vi "Dipper Fridge Resistance Measurement 1.3.vi"() -> ()   [LabVIEW 2011]
uses:
  <vilib>/express/express arith-compare/Formula/XNode/ExpressFormulaBlockNode.xnode
panel:
  out "He Pot Temperature":cluster{dbl[], dbl[]}(graph)
  out "Sample Resistance":dbl[][](graph)
  in  "Sample":bool
  out "Thermometer":bool
  out "Sample":bool
  in  "Timer":bool caption="Reset"
  out "Time Elapsed":string
  out "Output Power":dbl[unit]
  out "Heater Power (%)":string
  in  "Save":bool
  out "var":i32
  in  "error in (no error) 2":errorcluster
  in  "Output Range":string(combo)
  in  "Heater Power (%)":dbl caption="y"
  out "Heater Type (in Ohm)":string
  out "Heater Current (in %)":string
  out "Heater":bool
  in  "Heater":bool
  out "Boolean":bool
  in  "Power":bool
  in  "Date format (0)":enum16{"short", "long", "abbreviated"}(ring)
  out "Thermometer A":cluster{dbl[], dbl[unit][]}(graph)
  out "size (in bytes)":i64
  out "Thermometer (Ge17035)":cluster{dbl[], dbl[]}(graph)
  out "Warning":string="Can't be smaller than 1 s"
  in  "File Path":path
  out "current time":timestamp
  out "Number of Data points":i32
  in  "Time delay":u32=500 min=500 max=10000
  in  "error in (no error)":errorcluster
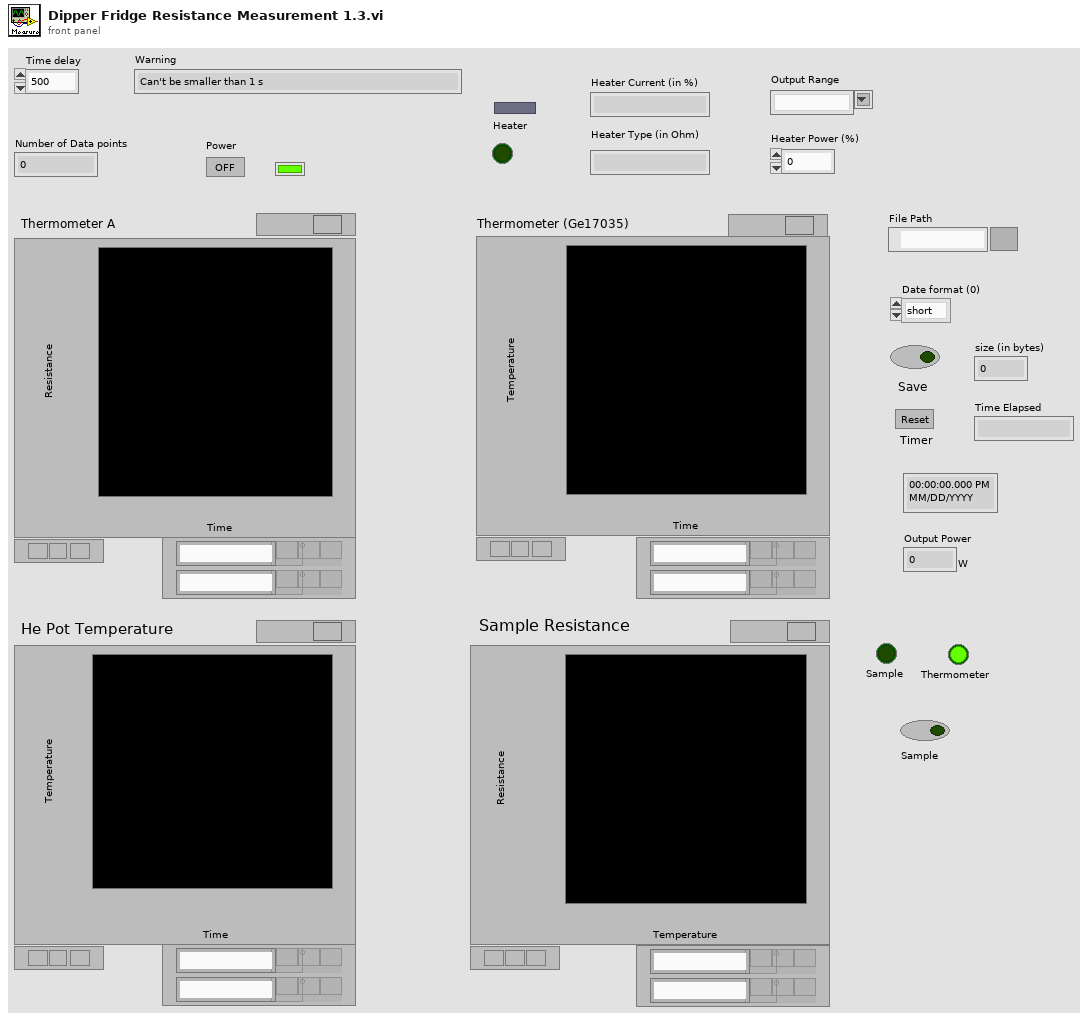
[diagram p1: front panel]
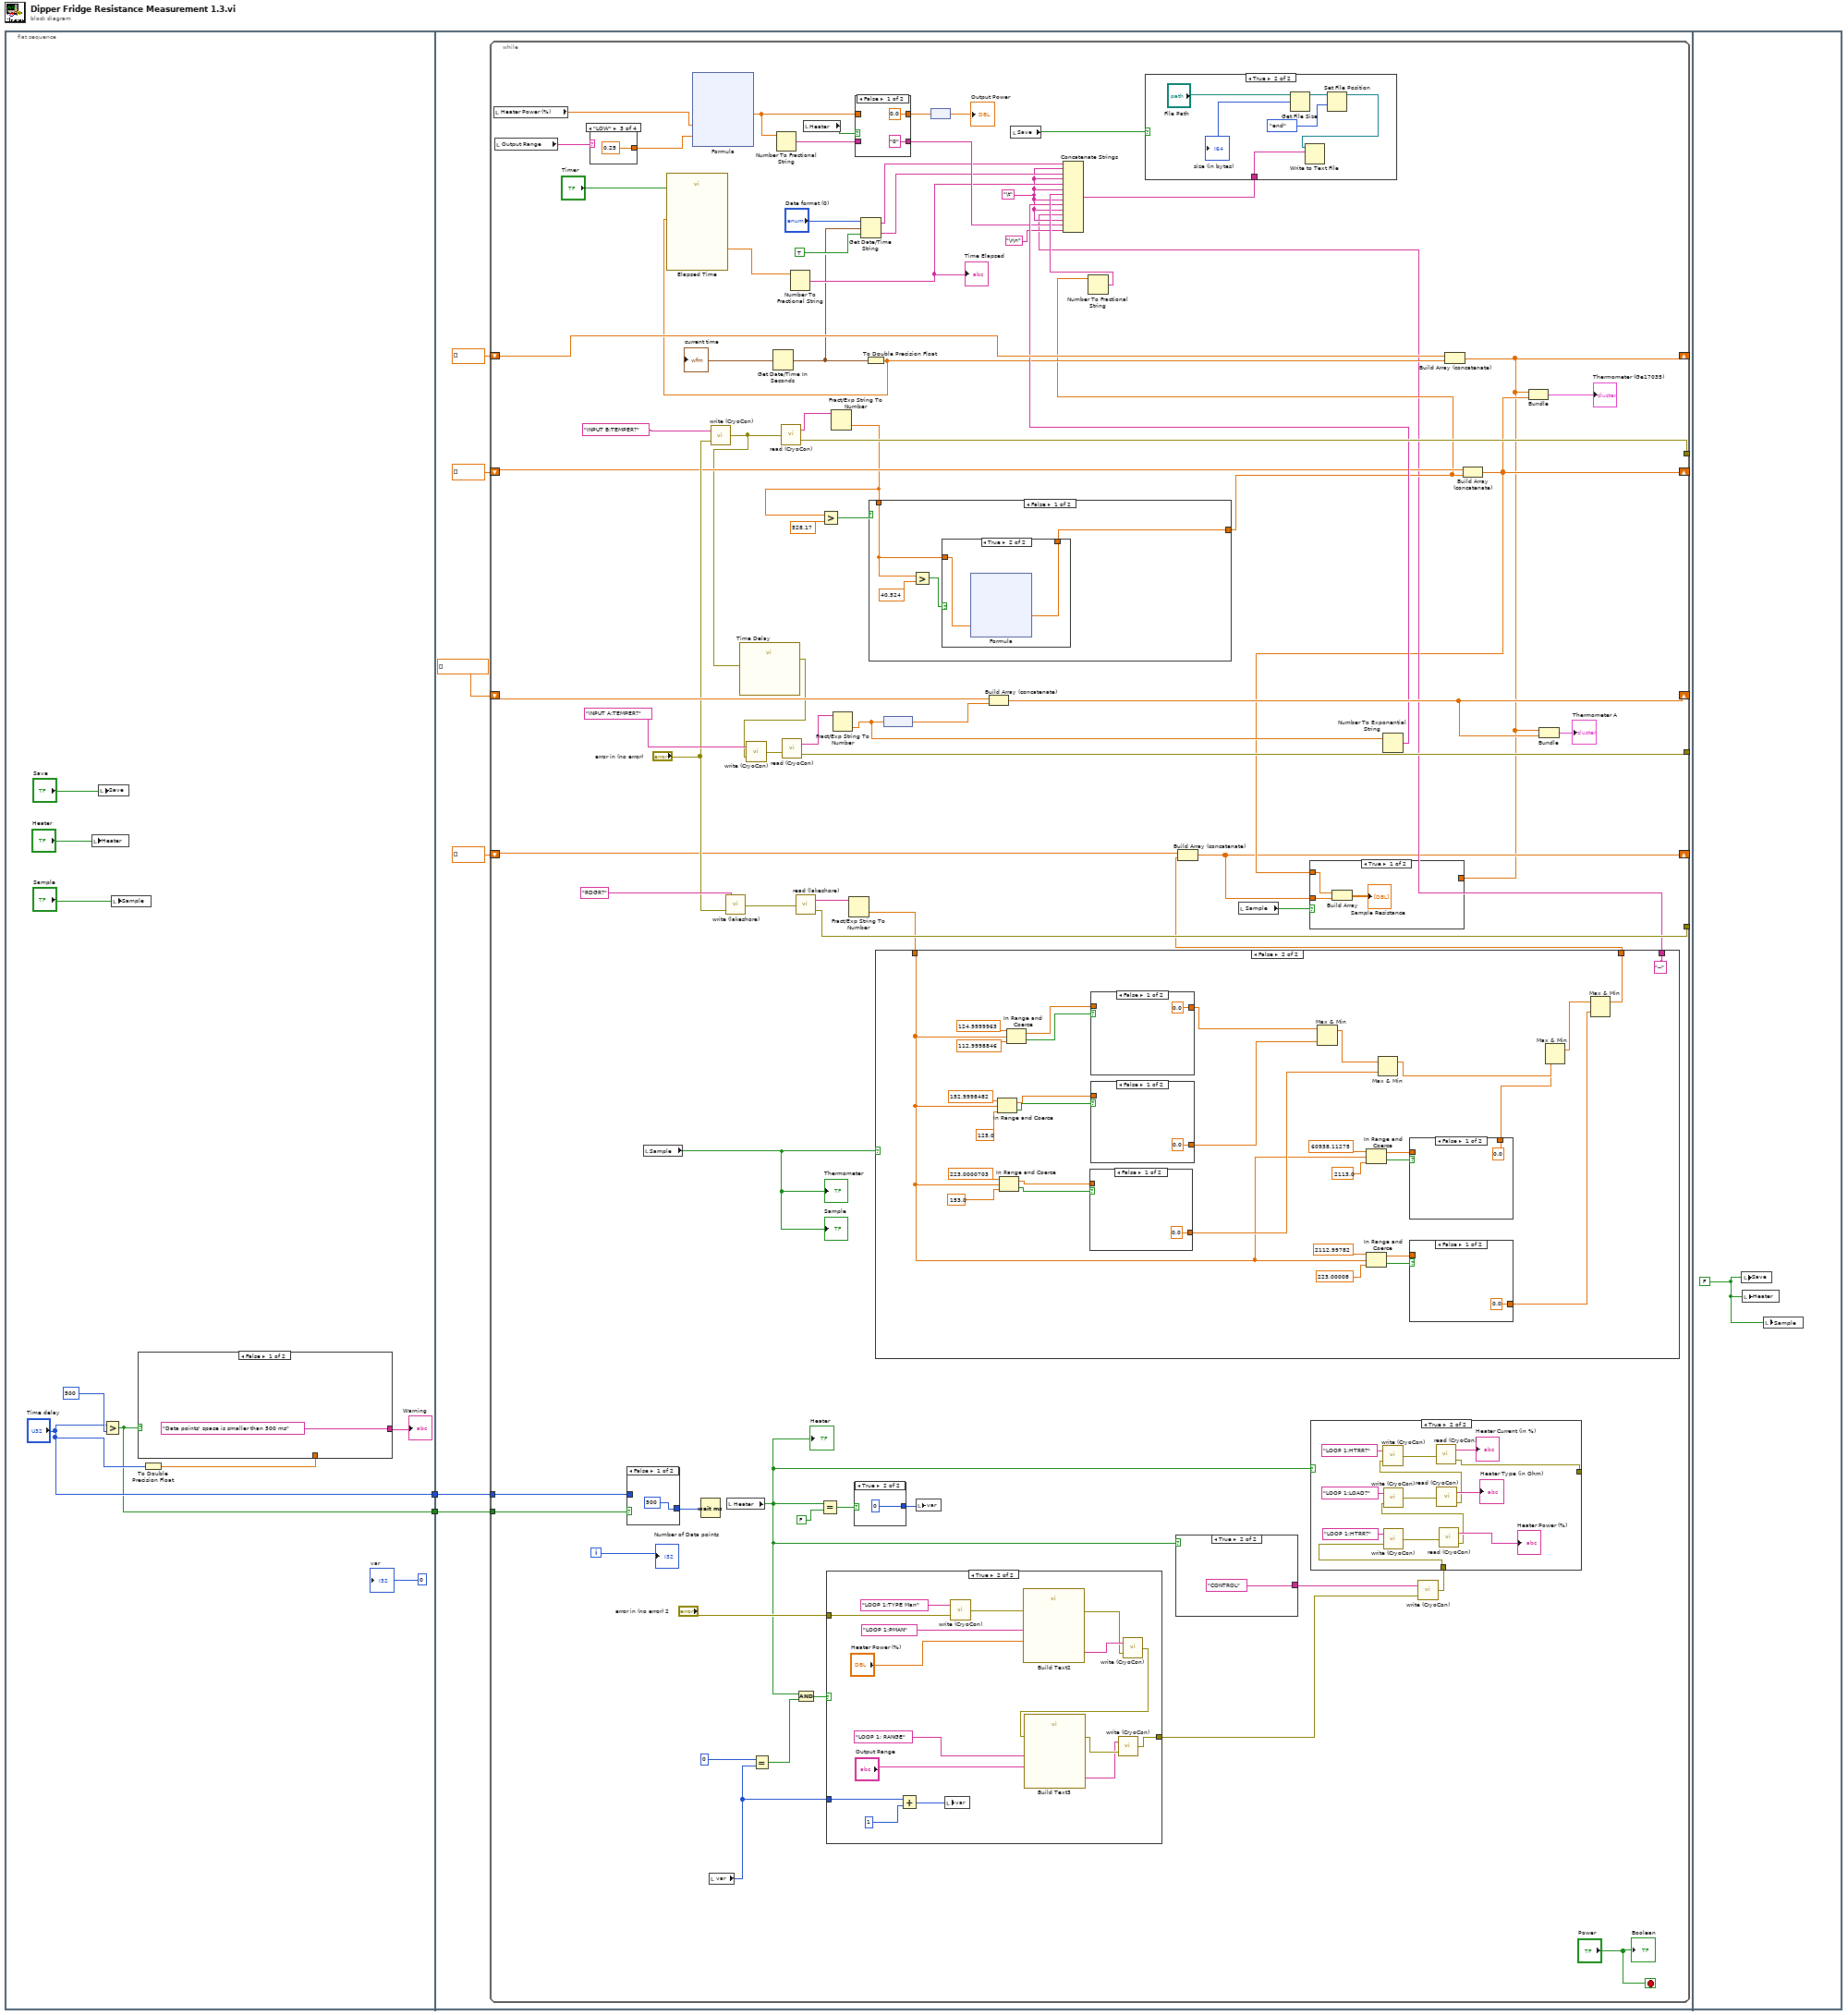
[diagram p0: block diagram]
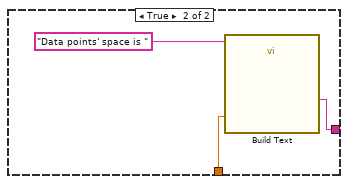
[diagram p2: hidden frame]
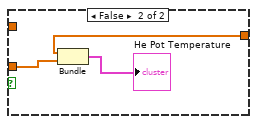
[diagram p3: hidden frame]
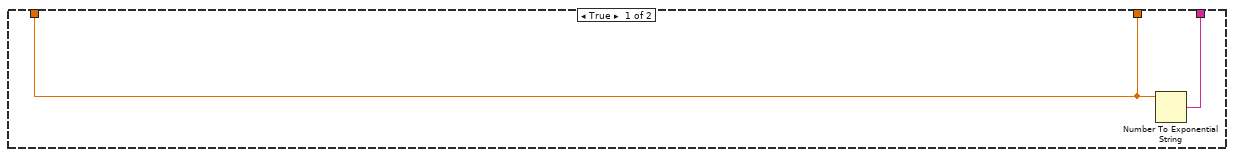
[diagram p4: hidden frame]
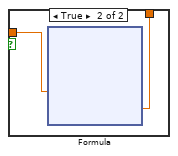
[diagram p5: hidden frame]
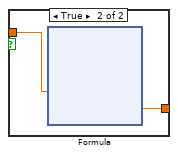
[diagram p6: hidden frame]
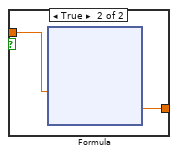
[diagram p7: hidden frame]
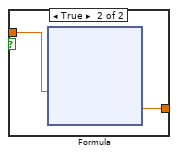
[diagram p8: hidden frame]
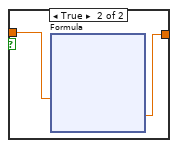
[diagram p9: hidden frame]
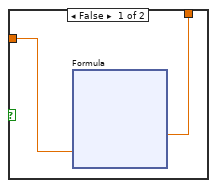
[diagram p10: hidden frame]
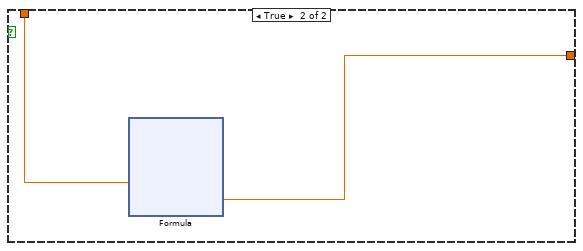
[diagram p11: hidden frame]
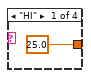
[diagram p13: hidden frame]
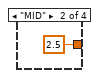
[diagram p14: hidden frame]
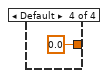
[diagram p15: hidden frame]
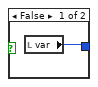
[diagram p16: hidden frame]
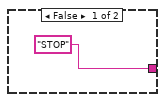
[diagram p19: hidden frame]
diagram:
  n1 = flat-sequence {
    tunnel: ["Time delay"] -> w2
    tunnel: [w6] -> w1
    tunnel: w2 -> [w21]
    tunnel: w1 -> [w20]
    frame #0 {
      n2 = local write "Heater"("Heater") -> ()
      n3 = local write "Save"("Save") -> ()
      n4 = Greater?(x="Time delay", y=u32 500 ("x")) -> (0:w6:bool)
      n5 = local write "Sample"("Sample") -> ()
      n6 = To Double Precision Float(number="Time delay") -> (double precision float=w8:dbl)
      n7 = case shown="False" w6 {
        tunnel: w8 -> [_ w13]
        tunnel: ["Data points' space is smaller than 500 ms" w15] -> w9
        frame False {
        }
        frame True {
          n8 = call "Build Text"("Beginning Text"="Data points' space is ", "Y"=w13) -> ("Result"=w15:string)  [unwired: 12 in, 1 out]
        }
      }
      "Warning" <- w9
      "var" <- 0 ("var")
    }
    frame #1 {
      n9 = while {
        tunnel: [w94] -> _
        tunnel: [w93] -> _
        tunnel: [w89] -> _
        shift-right: [w22] -> _
        shift-left: dbl[] [] -> [w84]
        tunnel: w21 -> [w83]
        tunnel: w20 -> [w82]
        shift-right: [w77] -> _
        shift-left: dbl[unit][] [] -> [w78]
        shift-right: [w24] -> _
        shift-left: dbl[] [] -> [w70]
        shift-right: [w23] -> _
        shift-left: dbl[] [] -> [w27]
        i -> [w86]
        stop <- "Power" stop-if-true
        w35 = "\t"
        n10 = local read "Heater Power (%)"() -> (w54:dbl)
        n11 = local read "Output Range"() -> (w52:string)
        n12 = case shown="\"LOW\"" w52 {
          tunnel: [25.0 ("X2") 2.5 ("X2") 0.25 ("X2") 0.0 ("X2")] -> w53
          frame "HI" {
          }
          frame "MID" {
          }
          frame "LOW" {
          }
          frame Default {
          }
        }
        n13 = case shown="False" w82 {
          tunnel: w83 -> [_ w280]
          tunnel: [500 w280] -> w81
          frame False {
          }
          frame True {
          }
        }
        n14 = local read "Sample"() -> (w26:bool)
        "Sample" <- w26
        "Thermometer" <- w26
        n15 = xnode "Formula"("X1"=w54, "X2"=w53) -> ("Result"=w46:dbl)  [unwired: 1 in, 1 out]
        n16 = Wait (ms)(milliseconds to wait=w81) -> ()  [unwired: 1 out]
        n17 = local read "var"() -> (w64:i32)
        n18 = call "write (CryoCon).vi"("error in (no error)"="error in (no error)", "write buffer"="INPUT B:TEMPER?") -> ("error out"=w44:errorcluster)
        n19 = call "write (lakeshore).vi"("error in (no error)"="error in (no error)", "write buffer"="RDGR?") -> ("error out"=w88:errorcluster)
        n20 = local read "Heater"() -> (w55:bool)
        "Heater" <- w55
        n21 = call "Time Delay"("error in (no error)"=w44) -> ("error out"=w43:errorcluster)  [unwired: 10 in]
        n22 = call "write (CryoCon).vi"("error in (no error)"=w43, "write buffer"="INPUT A:TEMPER?") -> ("error out"=w95:errorcluster)
        n23 = Equal?(x=0, y=w64) -> (x = y?=w62:bool)
        n24 = Get Date/Time In Seconds() -> (seconds since 1Jan1904=w41:timestamp)
        "current time" <- w41
        n25 = Number To Fractional String(number=w46) -> (F-format string=w50:string)  [unwired: 3 in]
        n26 = call "read (CryoCon).vi"("error in (no error)"=w44) -> ("read buffer"=w91:string, "error out"=w93:errorcluster)
        n27 = call "read (CryoCon).vi"("error in (no error)"=w95) -> ("read buffer"=w92:string, "error out"=w94:errorcluster)
        n28 = call "read (lakeshore).vi"("error in (no error)"=w88) -> ("read buffer"=w90:string, "error out"=w89:errorcluster)
        n29 = And(x=w55, y=w62) -> (x .and. y?=w61:bool)
        n30 = local read "Heater"() -> (w48:bool)
        n31 = Equal?(x=w55, y=FALSE ("Heater")) -> (x = y?=w57:bool)
        n32 = case shown="True" w61 {
          tunnel: [w246 w247] -> w60
          tunnel: "error in (no error) 2" -> [w246 w256]
          tunnel: w64 -> [_ w259]
          frame False {
          }
          frame True {
            n33 = Add(x=w259, y=1) -> (x+y=w257:i32)
            n34 = local write "var"(w257) -> ()
            n35 = call "write (CryoCon).vi"("error in (no error)"=w256, "write buffer"="LOOP 1:TYPE Man") -> ("error out"=w255:errorcluster)
            n36 = call "Build Text2"("x"="LOOP 1:PMAN" ("write buffer"), "y"="Heater Power (%)", "error in (no error)"=w255) -> ("Result"=w252:string, "error out"=w251:errorcluster)  [unwired: 11 in]
            n37 = call "write (CryoCon).vi"("error in (no error)"=w251, "write buffer"=w252) -> ("error out"=w250:errorcluster)
            n38 = call "Build Text3"("x"="LOOP 1: RANGE" ("write buffer"), "y"="Output Range", "error in (no error)"=w250) -> ("Result"=w248:string, "error out"=w249:errorcluster)  [unwired: 11 in]
            n39 = call "write (CryoCon).vi"("error in (no error)"=w249, "write buffer"=w248) -> ("error out"=w247:errorcluster)
          }
        }
        n40 = Fract/Exp String To Number(string=w91) -> (number=w32:dbl)  [unwired: 3 in, 1 out]
        n41 = Greater?(x=w32, y=528.17) -> (0:w33:bool)
        n42 = Fract/Exp String To Number(string=w92) -> (number=w74:dbl)  [unwired: 3 in, 1 out]
        n43 = Fract/Exp String To Number(string=w90) -> (number=w29:dbl)  [unwired: 3 in, 1 out]
        n44 = case shown="True" w57 {
          tunnel: [w234 0] -> w56
          frame False {
            n45 = local read "var"() -> (w234:i32)
          }
          frame True {
          }
        }
        n46 = case shown="False" w48 {
          tunnel: w50 -> [_ w229]
          tunnel: ["0" w229] -> w49
          tunnel: w46 -> [_ w228]
          tunnel: [0.0 ("Result") w228] -> w45
          frame False {
          }
          frame True {
          }
        }
        n47 = Get Date/Time String(date format (0)="Date format (0)", seconds (now)=w41, want seconds? (F)=TRUE) -> (date string=w36:string, time string=w37:string)
        n48 = To Double Precision Float(number=w41) -> (double precision float=w39:dbl)
        n49 = call "Elapsed Time"("Reset"="Timer", "Set Start Time (s)"=w39) -> ("Elapsed Time (s)"=w40:dbl)  [unwired: 10 in, 7 out]
        n50 = Number To Fractional String(number=w40) -> (F-format string=w42:string)  [unwired: 3 in]
        "Time Elapsed" <- w42
        n51 = case shown="False" w33 {
          tunnel: w32 -> [w193 w217]
          tunnel: [w192 w216] -> w31
          frame False {
            n52 = Greater?(x=w193, y=40.524) -> (0:w194:bool)
            n53 = case shown="True" w194 {
              tunnel: [w197 w207] -> w192
              tunnel: w193 -> [w196 w206]
              frame False {
                n54 = xnode "Formula"("X1"=w196) -> ("Result"=w197:dbl)  [unwired: 1 in, 1 out]
              }
              frame True {
                n55 = xnode "Formula"("X1"=w206) -> ("Result"=w207:dbl)  [unwired: 1 in, 1 out]
              }
            }
          }
          frame True {
            n56 = xnode "Formula"("X1"=w217) -> ("Result"=w216:dbl)  [unwired: 1 in, 1 out]
          }
        }
        n57 = case shown="False" w26 {
          tunnel: [w105 "--"] -> w30
          tunnel: w29 -> [w104 w106]
          tunnel: [w104 w108] -> w28
          frame True {
            n58 = Number To Exponential String(number=w104) -> (E-format string=w105:string)  [unwired: 3 in]
          }
          frame False {
            n59 = In Range and Coerce(upper limit=152.9998482, x=w106, lower limit=125.0) -> (coerced(x)=w129:dbl, In Range?=w130:bool)
            n60 = In Range and Coerce(upper limit=223.0000703, x=w106, lower limit=153.0) -> (coerced(x)=w125:dbl, In Range?=w126:bool)
            n61 = In Range and Coerce(upper limit=124.9999963, x=w106, lower limit=112.9998846) -> (coerced(x)=w133:dbl, In Range?=w134:bool)
            n62 = case shown="False" w126 {
              tunnel: w125 -> [_ w161]
              tunnel: [0.0 ("Result") w160] -> w114
              frame False {
              }
              frame True {
                n63 = xnode "Formula"("X1"=w161) -> ("Result"=w160:dbl)  [unwired: 1 in, 1 out]
              }
            }
            n64 = case shown="False" w134 {
              tunnel: w133 -> [_ w183]
              tunnel: [0.0 ("Result") w182] -> w116
              frame False {
              }
              frame True {
                n65 = xnode "Formula"("X1"=w183) -> ("Result"=w182:dbl)  [unwired: 1 in, 1 out]
              }
            }
            n66 = case shown="False" w130 {
              tunnel: w129 -> [_ w172]
              tunnel: [0.0 ("Result") w171] -> w115
              frame False {
              }
              frame True {
                n67 = xnode "Formula"("X1"=w172) -> ("Result"=w171:dbl)  [unwired: 1 in, 1 out]
              }
            }
            n68 = Max & Min(x=w116, y=w115) -> (max(x,y)=w113:dbl)  [unwired: 1 out]
            n69 = In Range and Coerce(upper limit=60938.11275, x=w106, lower limit=2113.0) -> (coerced(x)=w117:dbl, In Range?=w118:bool)
            n70 = In Range and Coerce(upper limit=2112.99782, x=w106, lower limit=223.00008) -> (coerced(x)=w121:dbl, In Range?=w122:bool)
            n71 = Max & Min(x=w113, y=w114) -> (max(x,y)=w112:dbl)  [unwired: 1 out]
            n72 = case shown="False" w118 {
              tunnel: w117 -> [_ w139]
              tunnel: [0.0 ("Result") w138] -> w111
              frame False {
              }
              frame True {
                n73 = xnode "Formula"("X1"=w139) -> ("Result"=w138:dbl)  [unwired: 1 in, 1 out]
              }
            }
            n74 = case shown="False" w122 {
              tunnel: w121 -> [_ w150]
              tunnel: [0.0 ("Result") w149] -> w109
              frame False {
              }
              frame True {
                n75 = xnode "Formula"("X1"=w150) -> ("Result"=w149:dbl)  [unwired: 1 in, 1 out]
              }
            }
            n76 = Max & Min(x=w112, y=w111) -> (max(x,y)=w110:dbl)  [unwired: 1 out]
            n77 = Max & Min(x=w110, y=w109) -> (max(x,y)=w108:dbl)  [unwired: 1 out]
          }
        }
        n78 = node(w74) -> (w79:dbl[unit])
        n79 = local write "var"(w56) -> ()
        n80 = node(w45) -> (→"Output Power":dbl[unit])
        n81 = Build Array (concatenate)(w78, w79) -> (w77:dbl[unit][])
        n82 = local read "Save"() -> (w59:bool)
        n83 = Number To Fractional String(number=w31) -> (F-format string=w73:string)  [unwired: 3 in]
        n84 = case shown="True" w55 {
          tunnel: ["STOP" ("write buffer") "CONTROL" ("write buffer")] -> w67
          frame False {
          }
          frame True {
          }
        }
        n85 = Build Array (concatenate)(w27, w28) -> (w23:dbl[])
        n86 = local read "Sample"() -> (w25:bool)
        n87 = Number To Exponential String(number=w74) -> (E-format string=w72:string)  [unwired: 3 in]
        n88 = Concatenate Strings(w36, w35, w37, w35, w42, w35, w73, w35, w72, w35, w30, w35, w49, "\r\n") -> (w80:string)
        n89 = case shown="True" w59 {
          tunnel: w80 -> [_ w286]
          frame False {
          }
          frame True {
            n90 = Get File Size(file="File Path") -> (refnum out=w284:refnum<file>, size (in bytes)=→"size (in bytes)":i64)  [unwired: 1 in, 1 out]
            n91 = Set File Position(refnum=w284, from (0:start)=enum16{"start", "end", "current"}."end") -> (refnum out=w283:refnum<file>)  [unwired: 2 in, 1 out]
            n92 = Write to Text File(file (use dialog)=w283, text=w286) -> ()  [unwired: 2 in, 3 out]
          }
        }
        n93 = call "write (CryoCon).vi"("error in (no error)"=w60, "write buffer"=w67) -> ("error out"=w66:errorcluster)
        n94 = case shown="True" w55 {
          tunnel: [w263 w271] -> _
          tunnel: w66 -> [w263 w268]
          frame False {
          }
          frame True {
            n95 = call "write (CryoCon).vi"("error in (no error)"=w268, "write buffer"="LOOP 1:HTRR?") -> ("error out"=w267:errorcluster)
            n96 = call "read (CryoCon).vi"("error in (no error)"=w267) -> ("read buffer"=→"Heater Power (%)":string, "error out"=w266:errorcluster)
            n97 = call "write (CryoCon).vi"("error in (no error)"=w266, "write buffer"="LOOP 1:LOAD?") -> ("error out"=w265:errorcluster)
            n98 = call "read (CryoCon).vi"("error in (no error)"=w265) -> ("read buffer"=→"Heater Type (in Ohm)":string, "error out"=w264:errorcluster)
            n99 = call "write (CryoCon).vi"("error in (no error)"=w264, "write buffer"="LOOP 1:HTRR?") -> ("error out"=w276:errorcluster)
            n100 = call "read (CryoCon).vi"("error in (no error)"=w276) -> ("read buffer"=→"Heater Current (in %)":string, "error out"=w271:errorcluster)
          }
        }
        n101 = Build Array (concatenate)(w84, w39) -> (w22:dbl[])
        n102 = Build Array (concatenate)(w70, w31) -> (w24:dbl[])
        n103 = case shown="True" w25 {
          tunnel: w24 -> [w99 _]
          tunnel: w23 -> [w100 w103]
          tunnel: w22 -> [_ w102]
          frame True {
            n104 = Build Array(w99, w100) -> (→"Sample Resistance":dbl[][])
          }
          frame False {
            n105 = Bundle(w102, w103) -> (→"He Pot Temperature":cluster{dbl[], dbl[]})  [unwired: 1 in]
          }
        }
        n106 = Bundle(w22, w24) -> (→"Thermometer (Ge17035)":cluster{dbl[], dbl[]})  [unwired: 1 in]
        n107 = Bundle(w22, w77) -> (→"Thermometer A":cluster{dbl[], dbl[unit][]})  [unwired: 1 in]
        "Number of Data points" <- w86
        "Boolean" <- "Power"
      }
    }
    frame #2 {
      w287 = FALSE ("Save")
      n108 = local write "Save"(w287) -> ()
      n109 = local write "Heater"(w287) -> ()
      n110 = local write "Sample"(w287) -> ()
    }
  }
